vi "ma_SML Exponential Weighting (complex input).vi"(2 "reset?":bool, 3 "average size":dbl, 4 "x":cdb[](array[numeric]) format="%.2f") -> (0 "averaged sofar":dbl, 1 "y":cdb[](array[numeric]) format="%.2f")   [LabVIEW 2020, in "NI_MAPro.lvlib"]
uses:
  NI_MAPro.lvlib
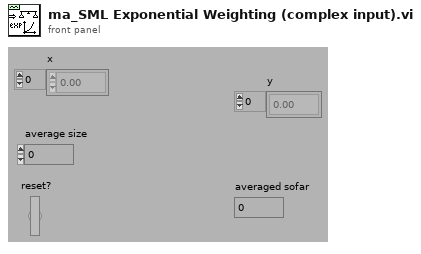
[diagram p1: front panel]
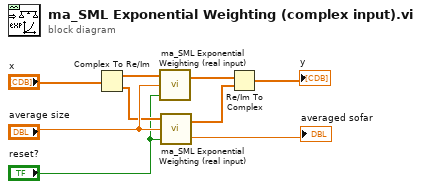
[diagram p0: block diagram]
diagram:
  n1 = Complex To Re/Im(x + iy="x") -> (x=w8:dbl[], y=w2:dbl[])
  n2 = call "ma_SML Exponential Weighting (real input).vi"("reset?"="reset?", "average size"="average size", "x"=w8) -> ("y"=w7:dbl[])  [unwired: 1 out]
  n3 = call "ma_SML Exponential Weighting (real input).vi"("reset?"="reset?", "average size"="average size", "x"=w2) -> ("averaged sofar"=→"averaged sofar":dbl, "y"=w5:dbl[])
  n4 = Re/Im To Complex(1:w5, 2:w7) -> (0:→"y":cdb[])
